vi "SPIKE-Microbit.vi"() -> ()   [LabVIEW 2016]
uses:
  VIs/uPythonX/uPythonX.xctl
panel:
  in  "read serial":T1(xcontrol)={"VISA Refnum in"="ASRL6::INSTR", "Python Code"="import pyb,utime\n\nuart = pyb.UART(1,9600, bits=8, parity=None, stop=1)\n\nwhile True:\n     if uart.any():\n          print(uart.readline())\n     utime.sleep(1)"}
  in  "LPF2Class":T1(xcontrol)={"VISA Refnum in"="ASRL5::INSTR", "Python Code"="import utime\nimport gc\nfrom microbit import *\n\nclass LPF2Class:\n     def __init__(self):\n          self.connected = False\n          self.tx = pin0\n          self.rx = pin1\n\n     def send_value(self, data):\n          value = (data & 0xFF)\n          payload = bytes([0xC0, value, 0xFF ^ 0xC0 ^ value])\n          size = uart.write(payload)\n          if not size:\n               self.connected = False\n\n     def initialize(self):\n          display.show(1)\n          self.tx.write_digital(0)\n          utime.sleep_ms(500)\n          self.tx.write_digital(1)\n          uart.init(baudrate=2400, bits=8, parity=None, stop=1,tx = pin0, rx = pin1)\n          uart.write(b'\\x00')\n          uart.write(b'\\x40\\x23\\x9C')  #CMD_TYPE (x40)  Type   checksum\n          uart.write(b'\\x49\\x00\\x00\\xB6')  #CMD_MODE (x49)  # Modes  # Views   checksum\n          uart.write(b'\\x52\\x00\\xC2\\x01\\x00\\x6E')  #CMD_SPEED (x52)  baud (LSB first)   checksum\n          uart.write(b'\\x5F\\x00\\x00\\x00\\x02\\x00\\x00\\x00\\x02\\xA0')  #CMD_VERSION (x5F)  Hardware_V  Software_V   checksum\n          uart.write(b'\\xA0\\x00\\x4C\\x50\\x46\\x32\\x2D\\x44\\x45\\x54\\x45\\x43\\x54\\x00\\x00\\x00\\x00\\x00\\x1D')  #CMD_INFO|bytes|mode  0 name 0   checksum\n          uart.write(b'\\x98\\x01\\x00\\x00\\x00\\x00\\x00\\x00\\x20\\x41\\x07')  #CMD_INFO|3|mode  1 (raw) raw_min  raw_max   checksum\n          uart.write(b'\\x98\\x02\\x00\\x00\\x00\\x00\\x00\\x00\\xC8\\x42\\xEF')  #CMD_INFO|3|mode  2 (pct) pct_min  pct_max   checksum\n          uart.write(b'\\x98\\x03\\x00\\x00\\x00\\x00\\x00\\x00\\x20\\x41\\x05')  #CMD_INFO|3|mode  3 (SI) si_min  si_max   checksum\n          uart.write(b'\\x80\\x04\\x00\\x7B')  #CMD_INFO|size|mode  0,4,symbol   checksum\n          uart.write(b'\\x88\\x05\\x10\\x00\\x62')  #CMD_INFO|1|mode  5 (FM) Function Map-In   -out   checksum\n          uart.write(b'\\x90\\x80\\x01\\x00\\x03\\x00\\xED')  #CMD_INFO|2|mode  x80 sample_size   Data_type   Figures   Decimals   checksum\n          utime.sleep_ms(5)\n          uart.write(b'\\x04') \n          display.show(4) \n          starttime = utime.ticks_ms()\n          currenttime = starttime\n          while (currenttime-starttime) < 2000:\n               utime.sleep_ms(5)\n               data = uart.read(uart.any())\n               if data.find(b'\\x04') >= 0:\n                    self.connected = True\n                    display.show(5) \n                    currenttime = starttime+3000 \n               else:\n                    self.connected = True\n                    currenttime = utime.ticks_ms()\n          self.tx.write_digital(0)\n          utime.sleep_ms(10)\n          uart.init(baudrate=115200, bits=8, parity=None, stop=1,tx = pin0, rx = pin1)\n          self.send_value(2)\ni = 0\nlpf2 = LPF2Class()\nlpf2.initialize()\n#display.show(lpf2.connected)\n\nwhile lpf2.connected:\n    lpf2.send_value(i)\n    i += 1\n    if i > 10: \n        i = 0\n    utime.sleep_ms(200)\n          "}
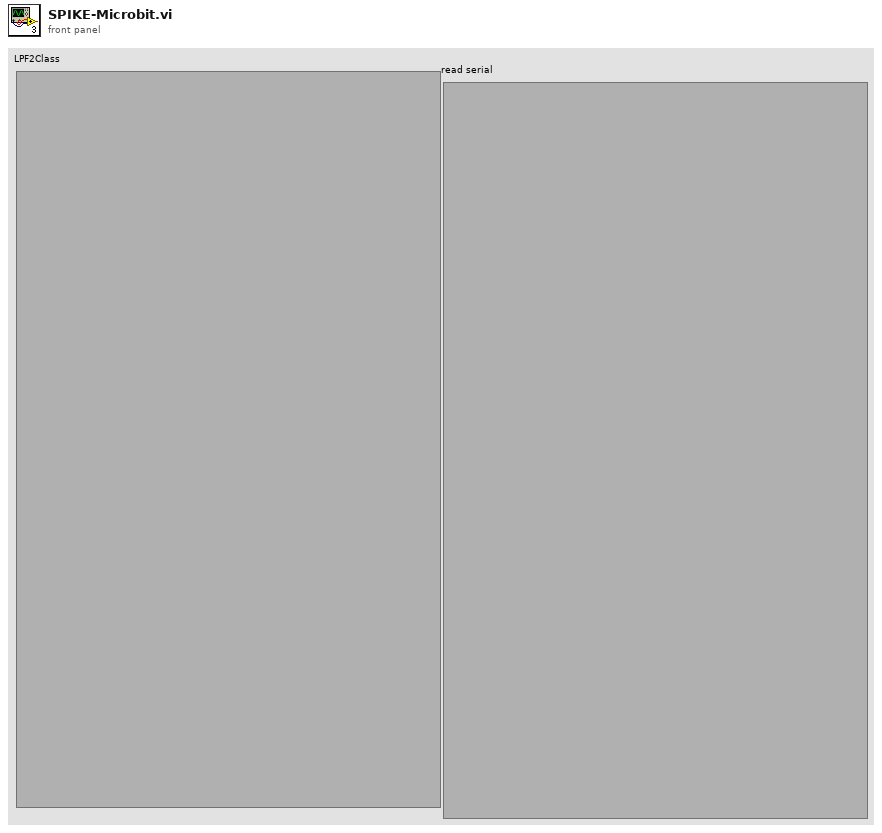
[diagram p1: front panel]
types:
  T1 = cluster{"VISA Refnum in":refnum<visa-resource-name>, "Python Code":string}
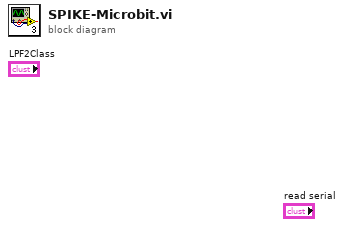
[diagram p0: block diagram]
diagram:
